vi "get status.vi"(8 "error in (no error)":errorcluster caption="entrée d'erreur (pas d'erreur)", 10 "status":u32, 11 "hHandle":i32) -> (0 "error out":errorcluster caption="sortie d'erreur", 2 "status out":u32)   [LabVIEW 2020, in "usb_relay_device.lvlib"]
doc: "int EXPORT_API usb_relay_device_get_status(int hHandle, unsigned int *status);"
uses:
  usb_relay_device.lvlib
  usb_relay_device.dll
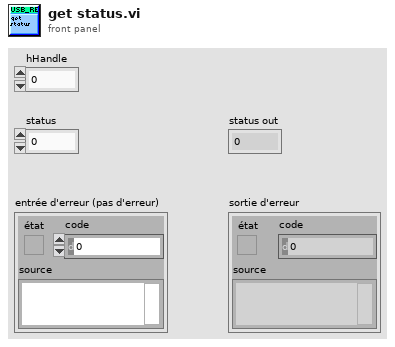
[diagram p1: front panel]
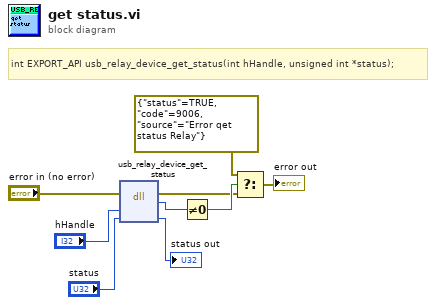
[diagram p0: block diagram]
diagram:
  # "int EXPORT_API usb_relay_device_get_status(int hHandle, unsigned int *status);"
  n1 = dll-call lib="C:/Users/ngarcin/OneDrive - Altyor/Standard TB/Class/Relay_Board/Relay_Board usb_Relay_device/usb_relay_device/usb_relay_device.dll" fn="usb_relay_device_get_status"(error in="error in (no error)", "hHandle"="hHandle", "status"="status") -> (error out=w2:errorcluster, "type de retour"=w1:i32, "status"=→"status out":u32)  [unwired: 3 in, 1 out]
  n2 = Not Equal To 0?(x=w1) -> (x != 0?=w5:bool)
  n3 = Select(t=errorcluster {"status"=TRUE, "code"=9006, "source"="Error qet status Relay"} ("sortie d'erreur"), s=w5, f=w2) -> (s? t:f=→"error out":errorcluster)
